vi "get_minimum_output_value.vi"(8 "error in (no error)":errorcluster, 11 "GenericWriteSignals.lvclass in":refnum<class "SignalWriterMH110203USBStepperMotor.lvclass">) -> (0 "error out":errorcluster, 2 "minimum output value":dbl, 3 "GenericWriteSignals.lvclass out":refnum<class "SignalWriterMH110203USBStepperMotor.lvclass">)   [LabVIEW 2010, in "SignalWriterMH110203USBStepperMotor.lvclass"]
uses:
  SignalWriterMH110203USBStepperMotor.lvclass
  SignalWriterMH110203USBStepperMotor.lvclass/SignalWriterMH110203USBStepperMotor.ctl
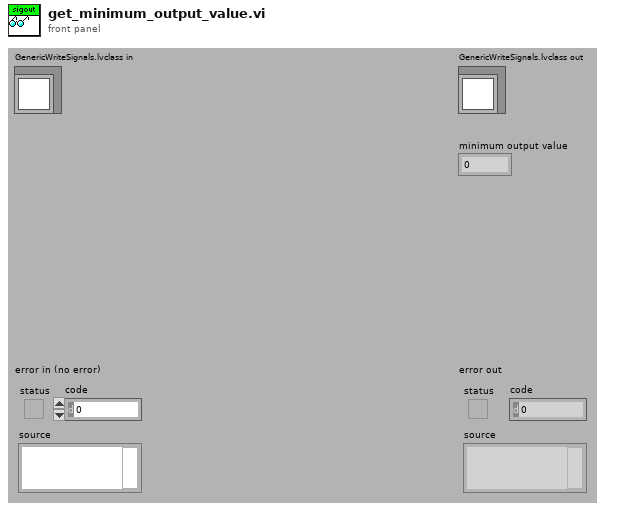
[diagram p1: front panel]
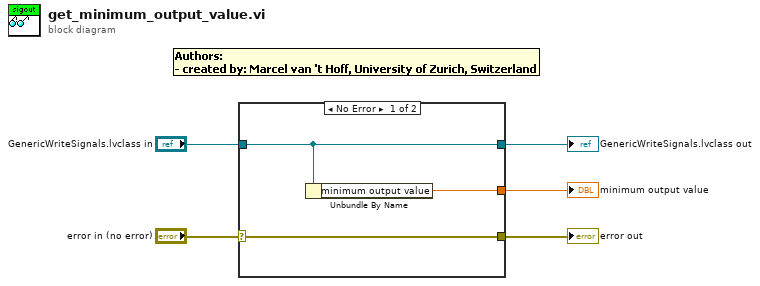
[diagram p0: block diagram]
diagram:
  n1 = case shown="No Error" "error in (no error)" {
    selector: "error in (no error)" -> [w8 w9]
    tunnel: [w8 w9] -> w3
    tunnel: [w7 w10] -> w2
    tunnel: "GenericWriteSignals.lvclass in" -> [w7 w10]
    tunnel: [w6 _] -> w1
    frame No Error {
      n2 = Unbundle By Name(w7) -> ("minimum output value"=w6:dbl)
    }
    frame Error {
    }
  }
  "error out" <- w3
  "GenericWriteSignals.lvclass out" <- w2
  "minimum output value" <- w1
